vi "Monitoring_receiver_v2.0.vi"() -> ()   [LabVIEW 2015, in "Monitoring_receiver.lvlib"]
doc: "Digital Receiver example.\n\nAuthor : Peter Vago NI SE, 2017 November\nLicense: ni.com/samplecodelicense"
uses:
  Monitoring_receiver.lvlib
  <userlib>/SE-APP-Receiver/NI5772/7976R_v1/7976R_v1.lvclass
  <vilib>/userdefined/High Color/nirio_resource_hc.ctl
panel:
  in  "enable.servers":bool
  out "Buffer status":u32(slide) scale=0.0..20000000.0
  in  "Channel IQ Rate (Hz)":dbl[](array[numeric])=[50500.0] format="%.2p"
  in  "Center Frequency (Hz)":dbl[](array[numeric])=[201000000.0] format="%_10f"
  out "ddc.number.of.ch":u8
  out "Fw Version":string="1.7.5"
  out "max value":i16
  out "cmd.received":string
  in  "Client Closed 2":string="The client VI closed the connection."
  out "cmd.server.ready":bool caption="TCP Cmd Srv Rdy"
  out "data.server.ready":bool caption="TCP Data Srv Rdy"
  in  "Client Closed":string="The client VI closed the connection."
  out "Power Spectrum":cluster{"f0":dbl, "df":dbl, "magnitude":dbl[]}[](graph)
  in  "Debug info":bool
  out "Tab Control":enum32{"Debug On", "Debug Off"}(tab)
  out "error out":errorcluster
  out "Remaining1":u32[](array[numeric])
  out "DMA \nTimed out":bool[](array[boolean])
  out "Device\nConfigured":bool[](array[boolean])
  in  "Resources":T1[](array[typedef])=["PXI1Slot6"]
  in  "Fetch Time (s)":dbl=0.01 format="%#.3p"
  in  "Continuous Acquisition":bool=TRUE
  in  "Software Trigger":bool
  out "Analog Input":waveform(dbl)[](graph) caption="Waveform"
  in  "stop":bool
  # "Digital Receiver Demo - NI 5772"
  # "Ver 3.0.0 , © Peter Vago, NI SE , 2017"
  # "Resources"
  # "Direct Digital Receiver"
  # "Debug Info"
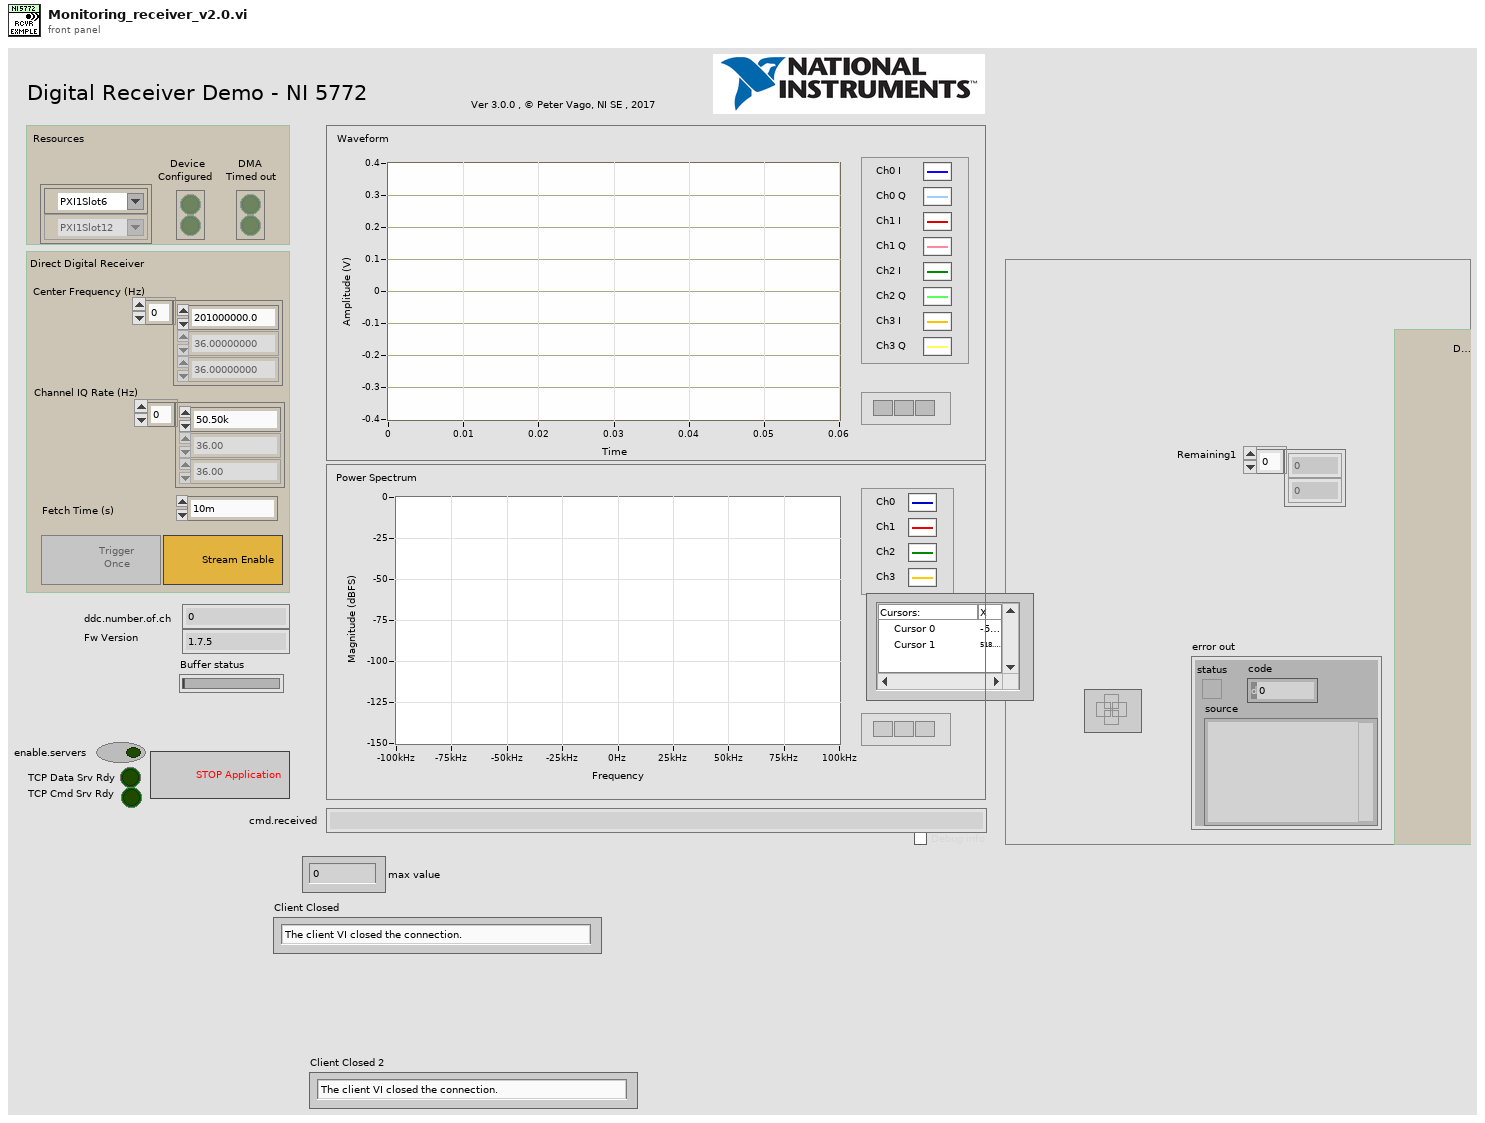
[diagram p1: front panel]
types:
  T1 = typedef "nirio_resource_hc.ctl" = tag
  T2 = enum16{"Normal mode", "TIS mode (CH0 only)", "TIS mode (CH1 only)"}
  T3 = enum8{"Internal Clock PLL Off", "Internal Clock PLL On (REF IN)", "External Clock (CLK_IN)", "Internal Clock PLL On (IoModSyncClk)"}
  T4 = cluster{"IQ Rate (Hz)":dbl[], "Freq Shift (Hz)":dbl[], "# of channels":u8, "Decimation factor":dbl[]}
  T5 = typedef "7976R_v1.lvclass/FPGA VI Reference_DDC_v1.8.ctl" = refnum<k20>
  T6 = cluster{"Bitfile Version":string, "FAM Configured":bool, "TIS Configured?":bool, "range (Vpp)":dbl, "Reference":T5}
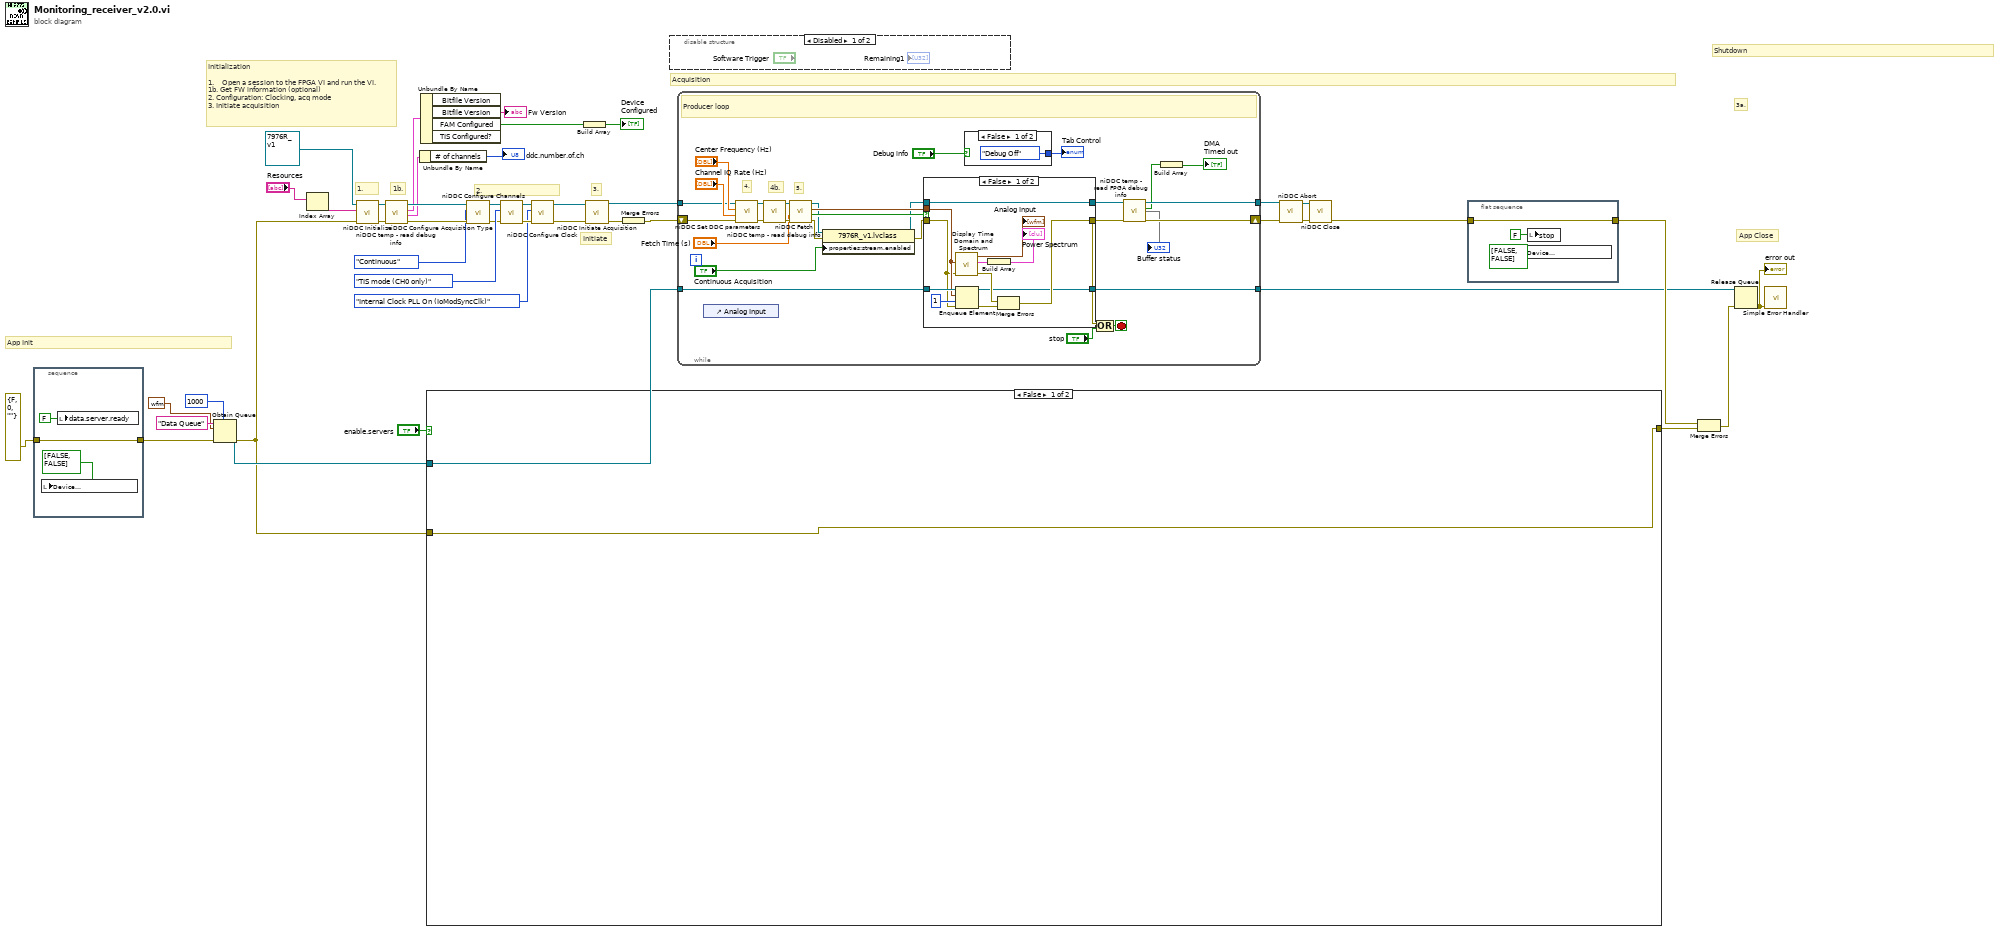
[diagram p0: block diagram]
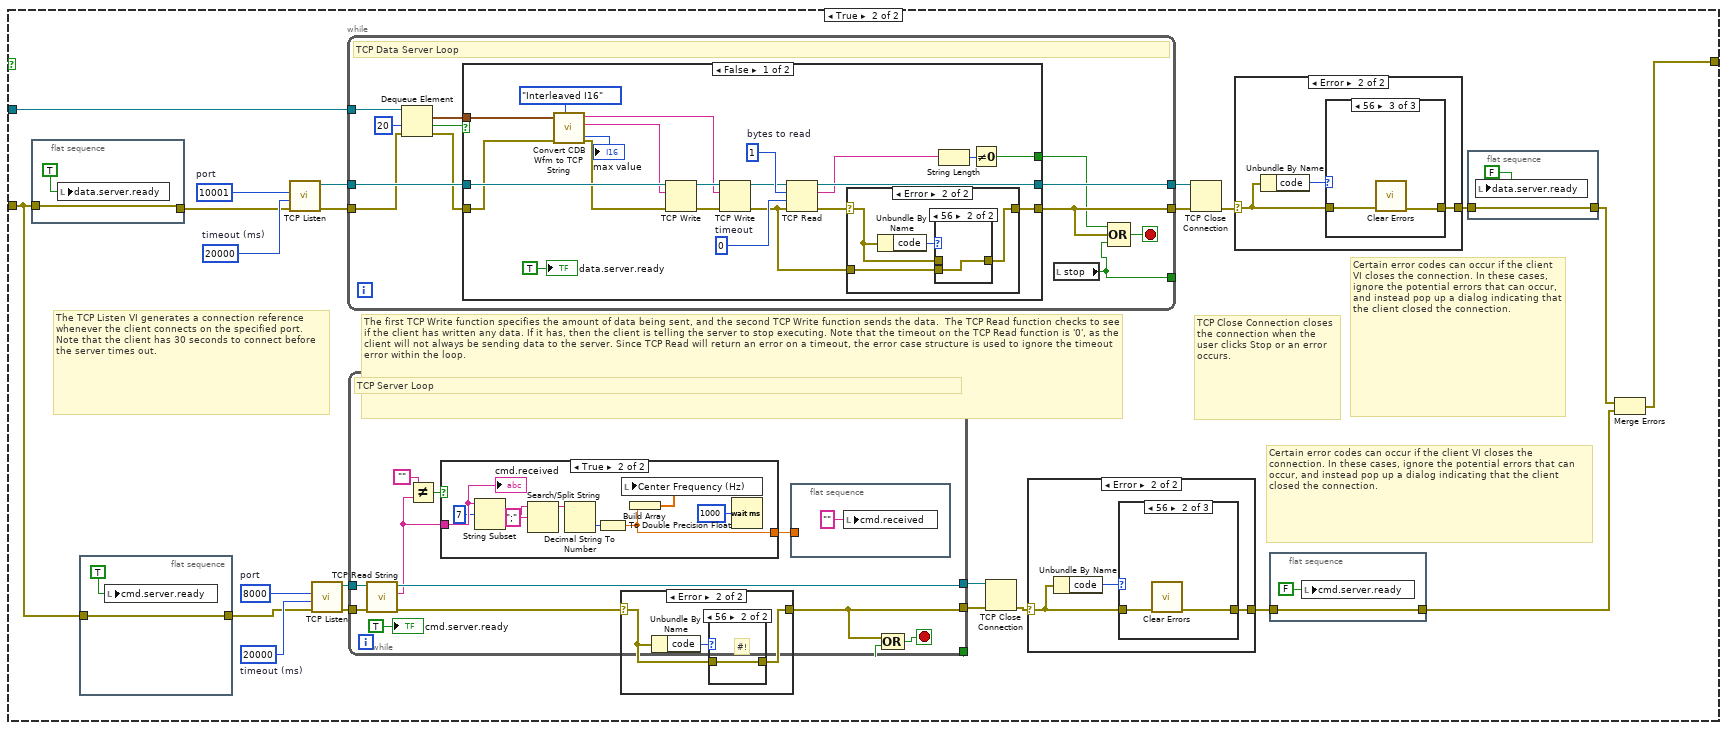
[diagram p2: hidden frame]
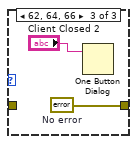
[diagram p5: hidden frame]
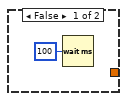
[diagram p6: hidden frame]
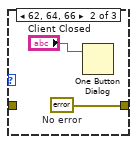
[diagram p11: hidden frame]
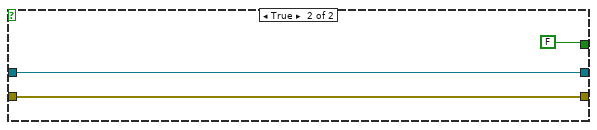
[diagram p14: hidden frame]
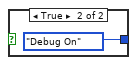
[diagram p16: hidden frame]
diagram:
  # "App Init"
  # "App Close"
  # "3."
  # "1b."
  # "1."
  # "2."
  # "Initiate"
  # "3a."
  # "Acquisition"
  # "Shutdown"
  # "Initialization\n\n1.    Open a session to the FPGA VI and run the VI.\n1b. Get FW information (optional)\n2. Configuration: Clocking, acq mode\n3. Initiate acquisition"
  n1 = stacked-sequence {
    tunnel: errorcluster {"status"=FALSE, "code"=0, "source"=""} ("error out") -> [w45]
    tunnel: [w45] -> w4
    frame #0 {
      n2 = local write "Device\nConfigured"(bool[] [FALSE, FALSE] ("Configured?")) -> ()
      n3 = local write "data.server.ready"(FALSE ("data.server.ready")) -> ()
    }
  }
  n4 = Obtain Queue(max queue size (-1, unlimited)=1000, name (unnamed)="Data Queue", element data type=waveform(cdb) {"t0"=timestamp(0 s since 1904-01-01), "dt"=1.0, "Y"=[]} ("output waveform"), error in (no error)=w4) -> (queue out=w41:refnum<queue>, error out=w3:errorcluster)  [unwired: 1 in, 1 out]
  n5 = Index Array(array="Resources") -> (element=w22:T1)  [unwired: 1 in]
  n6 = call-dynamic "niDDC Initialize.vi"("error in (no error)"=w3, "RIO0 Resource"=w22, "Class in"=refnum<class "7976R_v1.lvclass"> refnum ("Monitoring_receiver.lvlib:7976R_v1.lvclass")) -> ("error out"=w31:errorcluster, "Class out"=w32:refnum<class "7976R_v1.lvclass">)  [unwired: 7 in]
  n7 = call-dynamic "niDDC temp - read debug info.vi"("error in (no error)"=w31, "Class in"=w32) -> ("error out"=w27:errorcluster, "DDC"=w17:T4, "FPGA"=w18:T6, "Class out"=w28:refnum<class "7976R_v1.lvclass">)  [unwired: 6 in]
  n8 = Unbundle By Name(w17) -> ("# of channels"=→"ddc.number.of.ch":u8)
  n9 = Unbundle By Name(w18) -> ("Bitfile Version"=→"Fw Version":string, "FAM Configured"=w16:bool)  [unwired: 2 out]
  n10 = case shown="False" "enable.servers" {
    tunnel: w41 -> [_ w70]
    tunnel: [w47 w48] -> w38
    tunnel: w3 -> [w47 w51]
    frame False {
    }
    frame True {
      w54 = u16 8000  # port
      w55 = 20000  # timeout (ms)
      w63 = u16 10001  # port
      w64 = 20000  # timeout (ms)
      # "Certain error codes can occur if the client VI closes the connection. In these cases, ignore the potential errors that can occur, and instead pop up a dialog indicating that the client closed the connection."
      # "Certain error codes can occur if the client VI closes the connection. In these cases, ignore the potential errors that can occur, and instead pop up a dialog indicating that the client closed the connection."
      # "TCP Close Connection closes the connection when the user clicks Stop or an error occurs."
      # "The TCP Listen VI generates a connection reference whenever the client connects on the specified port. Note that the client has 30 seconds to connect before the server times out."
      # "The first TCP Write function specifies the amount of data being sent, and the second TCP Write function sends the data.  The TCP Read function checks to see if the client has written any data. If it has, then the client is telling the server to stop executing. Note that the timeout on the TCP Read function is '0', as the client will not always be sending data to the server. Since TCP Read will return an error on a timeout, the error case structure is used to ignore the timeout error within the loop."
      n11 = flat-sequence {
        tunnel: w51 -> [w113]
        tunnel: [w113] -> w61
        frame #0 {
          n12 = local write "data.server.ready"(TRUE ("data.server.ready")) -> ()
        }
      }
      n13 = flat-sequence {
        tunnel: w51 -> [w71]
        tunnel: [w71] -> w52
        frame #0 {
          n14 = local write "cmd.server.ready"(TRUE ("data.server.ready")) -> ()
        }
      }
      n15 = call <vilib>:"TCP Listen.vi"("error in (no error)"=w61, "timeout ms (wait forever: -1)"=w64, "port"=w63) -> ("error out"=w65:errorcluster, "connection ID"=w66:refnum<k5>)  [unwired: 4 in, 3 out]
      n16 = call <vilib>:"TCP Listen.vi"("error in (no error)"=w52, "timeout ms (wait forever: -1)"=w55, "port"=w54) -> ("error out"=w56:errorcluster, "connection ID"=w57:refnum<k5>)  [unwired: 4 in, 3 out]
      n17 = while {
        tunnel: [w134] -> w68
        tunnel: [w135] -> w69
        tunnel: w66 -> [w137]
        tunnel: w65 -> [w132]
        tunnel: w70 -> [w133]
        tunnel: [w127] -> _
        stop <- w136 stop-if-true
        # "TCP Data Server Loop"
        n18 = Dequeue Element(queue=w133, timeout in ms (-1)=20, error in (no error)=w132) -> (element=w128:waveform(cdb), timed out?=w130:bool, error out=w129:errorcluster)  [unwired: 1 out]
        n19 = case shown="False" w130 {
          tunnel: w137 -> [w158 w168]
          tunnel: [w151 w168] -> w135
          tunnel: [w147 FALSE] -> w126
          tunnel: [w145 w167] -> w134
          tunnel: w129 -> [w141 w167]
          tunnel: w128 -> [w142 _]
          frame False {
            w150 = 0  # timeout
            w153 = 1  # bytes to read
            n20 = call "Convert CDB Wfm to TCP String.vi"("Format (Intlvd I16)"=enum16{"Interleaved I16", "Interleaved DBL"}."Interleaved I16", "error in (no error)"=w141, "CDB Wfm in"=w142) -> ("error out"=w140:errorcluster, "Message size"=w155:string, "TCP message"=w154:string, "max value"=→"max value":i16)  [unwired: 5 in]
            n21 = TCP Write(connection ID=w158, data in=w155, error in (no error)=w140) -> (connection ID out=w157:refnum<k5>, error out=w156:errorcluster)  [unwired: 2 out]
            n22 = TCP Write(connection ID=w157, data in=w154, error in (no error)=w156) -> (connection ID out=w152:refnum<k5>, error out=w144:errorcluster)  [unwired: 2 out]
            n23 = TCP Read(connection ID=w152, bytes to read=w153, error in (no error)=w144, 9:w150) -> (connection ID out=w151:refnum<k5>, data out=w148:string, error out=w146:errorcluster)  [unwired: 1 out]
            n24 = case shown="Error" w146 {
              selector: w146 -> [w159 w162]
              tunnel: [w159 w160] -> w145
              tunnel: w144 -> [_ w161]
              frame No Error {
              }
              frame Error {
                n25 = Unbundle By Name(w162) -> ("code"=w163:i32)
                n26 = case shown="56" w163 {
                  tunnel: w162 -> [w164 _]
                  tunnel: w161 -> [_ w165]
                  tunnel: [w164 w165] -> w160
                  frame Default {
                  }
                  frame 56 {
                  }
                }
              }
            }
            n27 = String Length(string=w148) -> (length=w149:i32)
            n28 = Not Equal To 0?(x=w149) -> (x != 0?=w147:bool)
            "data.server.ready" <- TRUE ("data.server.ready")
          }
          frame True {
          }
        }
        n29 = local read "stop"() -> (w127:bool)
        n30 = Compound Arithmetic op=OR(w126, w134, w127) -> (w136:bool)
      }
      n31 = while {
        tunnel: [w94] -> w59
        tunnel: [w88] -> w60
        tunnel: w57 -> [w91]
        tunnel: w56 -> [w92]
        tunnel: [w93] -> _
        stop <- w95 stop-if-true
        # "TCP Server Loop"
        n32 = call <vilib>:"TCP Read String.vi"("error in (no error)"=w92, "connection ID"=w91) -> ("error out"=w87:errorcluster, "data out"=w85:string, "connection ID out"=w88:refnum<k5>)  [unwired: 7 in]
        n33 = Not Equal?(x="", y=w85) -> (x != y?=w86:bool)
        n34 = case shown="True" w86 {
          tunnel: w85 -> [_ w106]
          tunnel: [_ w99] -> w84
          frame False {
            n35 = Wait (ms)(milliseconds to wait=u32 100) -> ()  [unwired: 1 out]
          }
          frame True {
            n36 = String Subset(string=w106, offset (0)=7) -> (substring=w104:string)  [unwired: 1 in]
            n37 = Search/Split String(string=w104, search string/char (-)=";") -> (substring before match=w102:string)  [unwired: 1 in, 2 out]
            n38 = Decimal String To Number(string=w102) -> (number=w101:i32)  [unwired: 2 in, 1 out]
            n39 = To Double Precision Float(number=w101) -> (double precision float=w99:dbl)
            n40 = Build Array(w99) -> (w98:dbl[])
            n41 = local write "Center Frequency (Hz)"(w98) -> ()
            n42 = Wait (ms)(milliseconds to wait=u32 1000) -> ()  [unwired: 1 out]
            "cmd.received" <- w106
          }
        }
        n43 = case shown="Error" w87 {
          selector: w87 -> [w107 w109]
          tunnel: [w107 w108] -> w94
          frame No Error {
          }
          frame Error {
            n44 = Unbundle By Name(w109) -> ("code"=w110:i32)
            n45 = case shown="56" w110 {
              tunnel: w109 -> [w111 w112]
              tunnel: [w111 w112] -> w108
              frame Default {
              }
              frame 56 {
                # "#!"
              }
            }
          }
        }
        n46 = flat-sequence {
          tunnel: w84 -> [_]
          frame #0 {
            n47 = local write "cmd.received"("" ("cmd.received")) -> ()
          }
        }
        n48 = local read "stop"() -> (w93:bool)
        n49 = Compound Arithmetic op=OR(w94, w93) -> (w95:bool)
        "cmd.server.ready" <- TRUE ("data.server.ready")
      }
      n50 = TCP Close Connection(connection ID=w60, error in (no error)=w59) -> (error out=w58:errorcluster)  [unwired: 2 out]
      n51 = case shown="Error" w58 {
        selector: w58 -> [w75 w77]
        tunnel: [w75 w76] -> w53
        frame No Error {
        }
        frame Error {
          n52 = Unbundle By Name(w77) -> ("code"=w78:i32)
          n53 = case shown="56" w78 {
            tunnel: w77 -> [w79 w81 _]
            tunnel: [w79 w80 w83] -> w76
            frame Default {
            }
            frame 56 {
              n54 = call <vilib>:"Clear Errors.vi"("error in (no error)"=w81) -> ("error out"=w80:errorcluster)  [unwired: 5 in, 1 out]
            }
            frame 62, 64, 66 {
              w83 = errorcluster {"status"=FALSE, "code"=0, "source"=""}  # No error
              n55 = One Button Dialog(message="Client Closed 2") -> ()  [unwired: 1 in, 1 out]
            }
          }
        }
      }
      n56 = TCP Close Connection(connection ID=w69, error in (no error)=w68) -> (error out=w67:errorcluster)  [unwired: 2 out]
      n57 = case shown="Error" w67 {
        selector: w67 -> [w117 w119]
        tunnel: [w117 w118] -> w62
        frame No Error {
        }
        frame Error {
          n58 = Unbundle By Name(w119) -> ("code"=w120:i32)
          n59 = case shown="56" w120 {
            tunnel: w119 -> [w121 _ w125]
            tunnel: [w121 w123 w124] -> w118
            frame Default {
            }
            frame 62, 64, 66 {
              w123 = errorcluster {"status"=FALSE, "code"=0, "source"=""}  # No error
              n60 = One Button Dialog(message="Client Closed") -> ()  [unwired: 1 in, 1 out]
            }
            frame 56 {
              n61 = call <vilib>:"Clear Errors.vi"("error in (no error)"=w125) -> ("error out"=w124:errorcluster)  [unwired: 5 in, 1 out]
            }
          }
        }
      }
      n62 = flat-sequence {
        tunnel: w53 -> [w73]
        tunnel: [w73] -> w50
        frame #0 {
          n63 = local write "cmd.server.ready"(FALSE ("data.server.ready")) -> ()
        }
      }
      n64 = flat-sequence {
        tunnel: w62 -> [w115]
        tunnel: [w115] -> w49
        frame #0 {
          n65 = local write "data.server.ready"(FALSE ("data.server.ready")) -> ()
        }
      }
      n66 = Merge Errors(w49, w50) -> (w48:errorcluster)
    }
  }
  n67 = call-dynamic "niDDC Configure Acquisition Type.vi"("error in (no error)"=w27, "Type"=enum16{"Continuous", "Finite"}."Continuous", "Class in"=w28) -> ("error out"=w25:errorcluster, "Class out"=w26:refnum<class "7976R_v1.lvclass">)  [unwired: 7 in]
  n68 = call-dynamic "niDDC Configure Channels.vi"("error in (no error)"=w25, "mode"=T2."TIS mode (CH0 only)", "Class in"=w26) -> ("error out"=w34:errorcluster, "Class out"=w35:refnum<class "7976R_v1.lvclass">)  [unwired: 7 in]
  n69 = call-dynamic "niDDC Configure Clock.vi"("error in (no error)"=w34, "Clock Source"=T3."Internal Clock PLL On (IoModSyncClk)", "Class in"=w35) -> ("error out"=w29:errorcluster, "Class out"=w30:refnum<class "7976R_v1.lvclass">)  [unwired: 7 in]
  n70 = Build Array(w16) -> (→"Device\nConfigured":bool[])
  n71 = call-dynamic "niDDC Initiate Acquisition.vi"("error in (no error)"=w29, "Class in"=w30) -> ("error out"=w14:errorcluster, "Class out"=w15:refnum<class "7976R_v1.lvclass">)  [unwired: 8 in]
  n72 = Merge Errors(w14) -> (w13:errorcluster)
  n73 = disable-structure shown="Disabled" {
    frame Disabled {
    }
    frame Enabled {
    }
  }
  n74 = while {
    shift-right: [w172] -> w8
    shift-left: w13 -> [w184]
    tunnel: [w173] -> w9
    tunnel: w41 -> [w193]
    tunnel: w15 -> [w186]
    tunnel: [w176] -> w6
    stop <- w196 stop-if-true
    # "4b."
    # "5."
    # "4."
    # "Producer loop"
    n75 = control-ref of="Analog Input"() -> ()  [unwired: 1 out]
    n76 = call-dynamic "niDDC Set DDC parameters.vi"("error in (no error)"=w184, "DDC IQ rates (Hz)"="Channel IQ Rate (Hz)", "DDC Freq shift (Hz)"="Center Frequency (Hz)", "Class in"=w186) -> ("error out"=w191:errorcluster, "Class out"=w192:refnum<class "7976R_v1.lvclass">)  [unwired: 6 in]
    n77 = call-dynamic "niDDC temp - read debug info.vi"("error in (no error)"=w191, "Class in"=w192) -> ("error out"=w189:errorcluster, "Class out"=w190:refnum<class "7976R_v1.lvclass">)  [unwired: 6 in, 2 out]
    n78 = call-dynamic "niDDC Fetch.vi"("error in (no error)"=w189, "seconds to read (-1:all)"="Fetch Time (s)", "Class in"=w190) -> ("error out"=w177:errorcluster, "Timeout?"=w183:bool, "Complex wfm out"=w182:waveform(cdb), "Class out"=w181:refnum<class "7976R_v1.lvclass">)  [unwired: 5 in]
    n79 = property class="7976R_v1.lvclass"(reference=w181, error in=w177, "properties:stream.enabled"="Continuous Acquisition") -> (reference out=w180:refnum<class "7976R_v1.lvclass">, error out=w178:errorcluster)
    n80 = case shown="False" w183 {
      tunnel: [w208 w213] -> w174
      tunnel: [w203 w214] -> w175
      tunnel: w180 -> [w203 w214]
      tunnel: w178 -> [w201 w213]
      tunnel: w193 -> [w211 w212]
      tunnel: w182 -> [w202 _]
      tunnel: [w200 w212] -> w176
      frame False {
        n81 = call "Display Time Domain and Spectrum.vi"("error in (no error)"=w201, "CDB Wfm in"=w202) -> ("error out"=w204:errorcluster, "Power Spectrum / PSD"=w206:cluster{"f0":dbl, "df":dbl, "magnitude":dbl[]}, "I and Q Waveform"=→"Analog Input":waveform(dbl)[])  [unwired: 7 in]
        n82 = Enqueue Element(queue=w211, element=w202, timeout in ms (-1)=1, error in (no error)=w201) -> (queue out=w200:refnum<queue>, error out=w209:errorcluster)  [unwired: 1 out]
        n83 = Build Array(w206) -> (→"Power Spectrum":cluster{"f0":dbl, "df":dbl, "magnitude":dbl[]}[])
        n84 = Merge Errors(w204, w209) -> (w208:errorcluster)
      }
      frame True {
      }
    }
    n85 = case shown="False" "Debug info" {
      tunnel: [enum32{"Debug On", "Debug Off"}."Debug Off" ("Tab Control") enum32{"Debug On", "Debug Off"}."Debug On" ("Tab Control")] -> w194
      frame False {
      }
      frame True {
      }
    }
    "Tab Control" <- w194
    n86 = Compound Arithmetic op=OR(w174, "stop") -> (w196:bool)
    n87 = call-dynamic "niDDC temp - read FPGA debug info.vi"("error in (no error)"=w174, "Class in"=w175) -> ("error out"=w172:errorcluster, "dma.overflow"=w171:bool, "Class out"=w173:refnum<class "7976R_v1.lvclass">, 4:→"Buffer status")  [unwired: 5 in, 1 out]
    n88 = Build Array(w171) -> (→"DMA \nTimed out":bool[])
  }
  n89 = call-dynamic "niDDC Abort.vi"("error in (no error)"=w8, "Class in"=w9) -> ("error out"=w10:errorcluster, "Class out"=w11:refnum<class "7976R_v1.lvclass">)  [unwired: 8 in]
  n90 = call-dynamic "niDDC Close.vi"("error in (no error)"=w10, "Class in"=w11) -> ("error out"=w7:errorcluster)  [unwired: 8 in, 1 out]
  n91 = flat-sequence {
    tunnel: w7 -> [w215]
    tunnel: [w215] -> w40
    frame #0 {
      n92 = local write "Device\nConfigured"(bool[] [FALSE, FALSE] ("Configured?")) -> ()
      n93 = local write "stop"(FALSE ("stop")) -> ()
    }
  }
  n94 = Merge Errors(w40, w38) -> (w39:errorcluster)
  n95 = Release Queue(queue=w6, error in (no error)=w39) -> (error out=w2:errorcluster)  [unwired: 1 in, 2 out]
  "error out" <- w2
  n96 = call <vilib>:"Simple Error Handler.vi"("error in (no error)"=w2) -> ()  [unwired: 4 in, 5 out]
